vi "Pulse.vi"(3 "Pulse Duration (ms)":u32=20, 4 "Trigger":bool, 5 "State In":bool) -> (2 "State Out":bool)   [LabVIEW 2018]
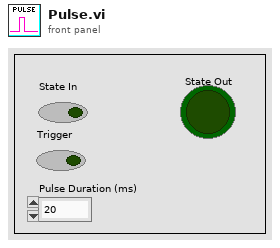
[diagram p1: front panel]
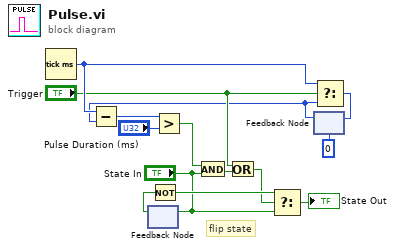
[diagram p0: block diagram]
diagram:
  # "flip state"
  n1 = Tick Count (ms)() -> (millisecond timer value=w14:u32)
  n2 = feedback #1() -> (w11:bool)  [unwired: 1 in]
  n3 = feedback-in #1("State In") -> ()
  n4 = Not(x=w11) -> (.not. x?=w12:bool)
  n5 = feedback #2(u32 0 ("millisecond timer value")) -> (w1:u32)
  n6 = Subtract(x=w14, y=w1) -> (x-y=w13:u32)
  n7 = Greater?(x=w13, y="Pulse Duration (ms)") -> (0:w9:bool)
  n8 = And(x=w9, y="State In") -> (x .and. y?=w6:bool)
  n9 = Or(x="Trigger", y=w6) -> (x .or. y?=w10:bool)
  n10 = Select(t=w12, s=w10, f="State In") -> (s? t:f=→"State Out":bool)
  n11 = Select(t=w14, s="Trigger", f=w1) -> (s? t:f=w3:u32)
  n12 = feedback-in #2(w3) -> ()
